vi "Amplitude.vi"(6 "Valid in":bool, 7 "Piezo setting":T1, 8 "Ch1 Q":fxp<+/-,32,14>, 9 "Ch1 I":fxp<+/-,32,14>, 10 "Ch0 Q":fxp<+/-,32,14>, 11 "Ch0 I":fxp<+/-,32,14>) -> (0 "output valid":bool, 3 "Ampl * dt":fxp<+/-,64,0>)   [LabVIEW 2018]
uses:
  Piezo setting.ctl
  <vilib>/rvi/FXPMathLib/FxpSqrt/subVIs/nifxpmath_Sqrt_SimConfig.ctl
  <vilib>/fxp/LVFixedPointOverflowPolicyTypeDef.ctl
  <vilib>/rvi/FXPMathLib/FxpSqrt/simVIs/DllSqrtTemp_sub.vi
  <vilib>/rvi/FXPMathLib/FxpSqrt/XNode/nifxpmath_Sqrt.xnode
  <vilib>/rvi/FXPMathLib/FxpMul/XNode/nifxpmath_Multiplier.xnode
  <vilib>/rvi/FXPMathLib/FxpAdd/XNode/nifxpmath_Add.xnode
  <vilib>/rvi/FXPMathLib/sim/FxpSim.dll
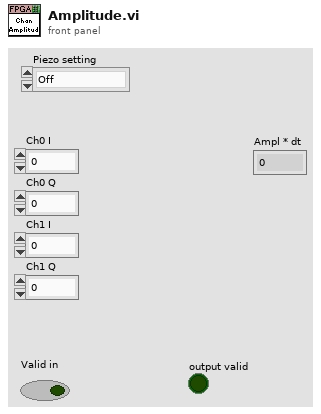
[diagram p1: front panel]
types:
  T1 = typedef "Piezo setting.ctl" = enum16{"Off", "On - Ch 0", "On - Ch 1"}
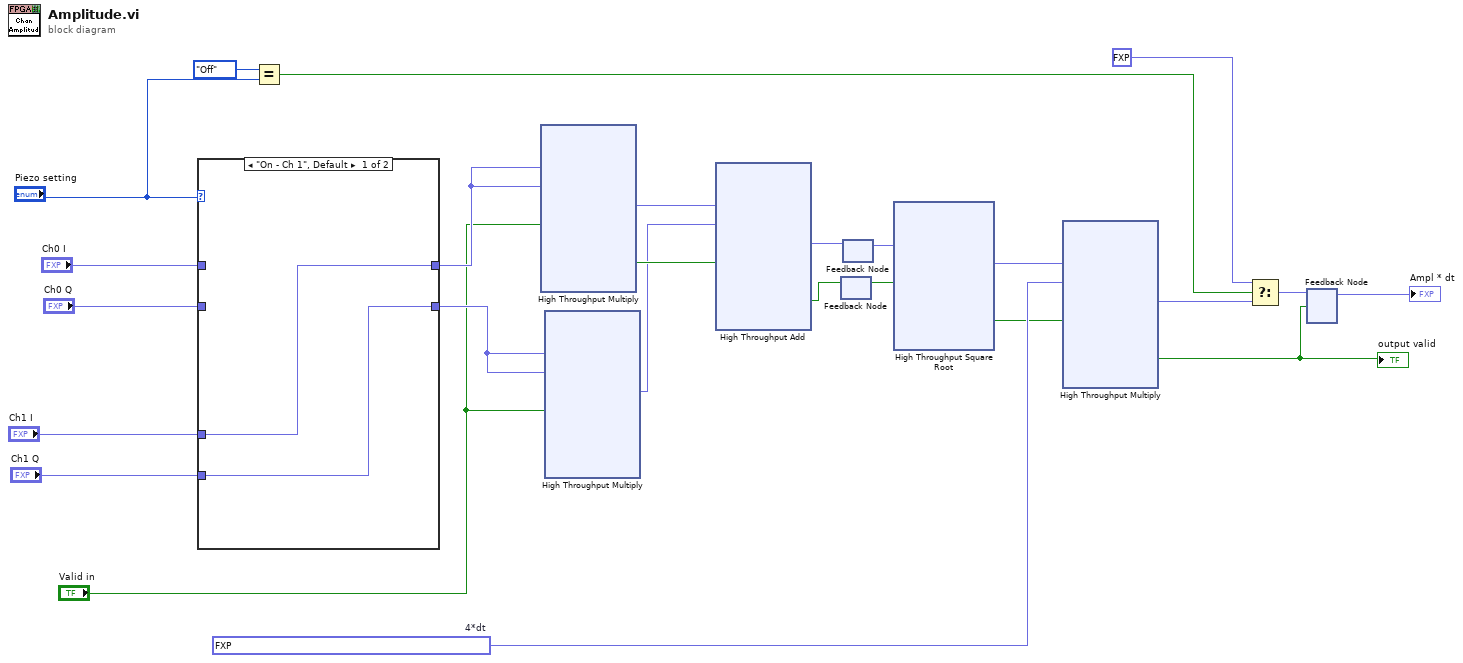
[diagram p0: block diagram]
diagram:
  w15 = fxp<+/-,33,-15> 4.000000011217253e-07  # 4*dt
  n1 = case shown="\"On - Ch 1\", Default" "Piezo setting" {
    tunnel: [w27 w29] -> w21
    tunnel: "Ch0 I" -> [_ w29]
    tunnel: [w26 w28] -> w18
    tunnel: "Ch0 Q" -> [_ w28]
    tunnel: "Ch1 I" -> [w27 _]
    tunnel: "Ch1 Q" -> [w26 _]
    frame "On - Ch 1", Default {
    }
    frame "On - Ch 0" {
    }
  }
  n2 = Equal?(x=Piezo_setting."Off", y="Piezo setting") -> (x = y?=w9:bool)
  n3 = xnode ("High Throughput Multiply")("x"=w21, "y"=w21, "input valid"="Valid in") -> ("x*y"=w20:fxp<+,64,28>, "output valid"=w19:bool)  [unwired: 1 in, 1 out]
  n4 = xnode ("High Throughput Multiply")("x"=w18, "y"=w18, "input valid"="Valid in") -> ("x*y"=w16:fxp<+,64,28>)  [unwired: 1 in, 2 out]
  n5 = xnode "High Throughput Add"("x"=w20, "y"=w16, "input valid"=w19) -> ("x+y"=w7:fxp<+,64,29>, "output valid"=w14:bool)  [unwired: 1 in, 1 out]
  n6 = feedback-in #1(w14) -> ()
  n7 = feedback #1() -> (w13:bool)  [unwired: 1 in]
  n8 = feedback #2() -> (w12:fxp<+,64,29>)  [unwired: 1 in]
  n9 = feedback-in #2(w7) -> ()
  n10 = xnode "High Throughput Square Root"("x"=w12, "input valid"=w13) -> ("sqrt(x)"=w5:fxp<+,33,15>, "output valid"=w4:bool)  [unwired: 1 in, 1 out]
  n11 = xnode ("High Throughput Multiply")("x"=w5, "y"=w15, "input valid"=w4) -> ("x*y"=w6:fxp<+/-,64,0>, "output valid"=w3:bool)  [unwired: 1 in, 1 out]
  "output valid" <- w3
  n12 = Select(t=fxp<+/-,64,0> 0.0, s=w9, f=w6) -> (s? t:f=w2:fxp<+/-,64,0>)
  n13 = feedback #3() -> (→"Ampl * dt":fxp<+/-,64,0>)  [unwired: 1 in]
  n14 = feedback-in #3(w2, w3) -> ()
